vi "Periodic Tasks.vi"(8 "error in":errorcluster) -> ()   [LabVIEW 2015]
doc: "This VI runs in parallel to other tasks. It can contain as many user-defined periodic loops as you need. These can carry out PID or other sorts of timed response."
uses:
  <vilib>/Rock Robotics/WPI/CAN/TalonSRX/WPI_CANTalonSRX_GlobalStatus.ctl
  <vilib>/Rock Robotics/Network Tables/NT Write Number.vi
  <vilib>/Rock Robotics/WPI/Solenoid/Deprecated/WPI_SolenoidSetBool.vi
  <vilib>/Rock Robotics/WPI/Solenoid/Deprecated/WPI_SolenoidGetBool.vi
panel:
  out "LowerRPM":dbl
  out "UpperRPM":dbl
  out "diff":dbl
  out "Talon SRX Status 2":T1
  out "Waveform Chart":cluster{dbl, dbl}(graph)
  in  "dT 2":dbl format="%#_13g"
  in  "I 2":dbl format="%#_13g"
  in  "P 2":dbl=1.0 format="%#_13g"
  in  "dT":dbl format="%#_13g"
  in  "I":dbl format="%#_13g"
  in  "P":dbl=1.0 format="%#_13g"
  out "Talon SRX Status":T1
  out "x/y":dbl=2.0599363125
  out "Shot":bool=TRUE
  in  "Left Art":dbl=0.5 format="%#_13g"
  in  "Right Art":dbl=0.5 format="%#_13g"
  in  "velocity_lower":dbl=1.0 format="%#_13g"
  in  "velocity_upper":dbl=1.0 format="%#_13g"
  out "error out":errorcluster
  # "change in time in milliseconds"
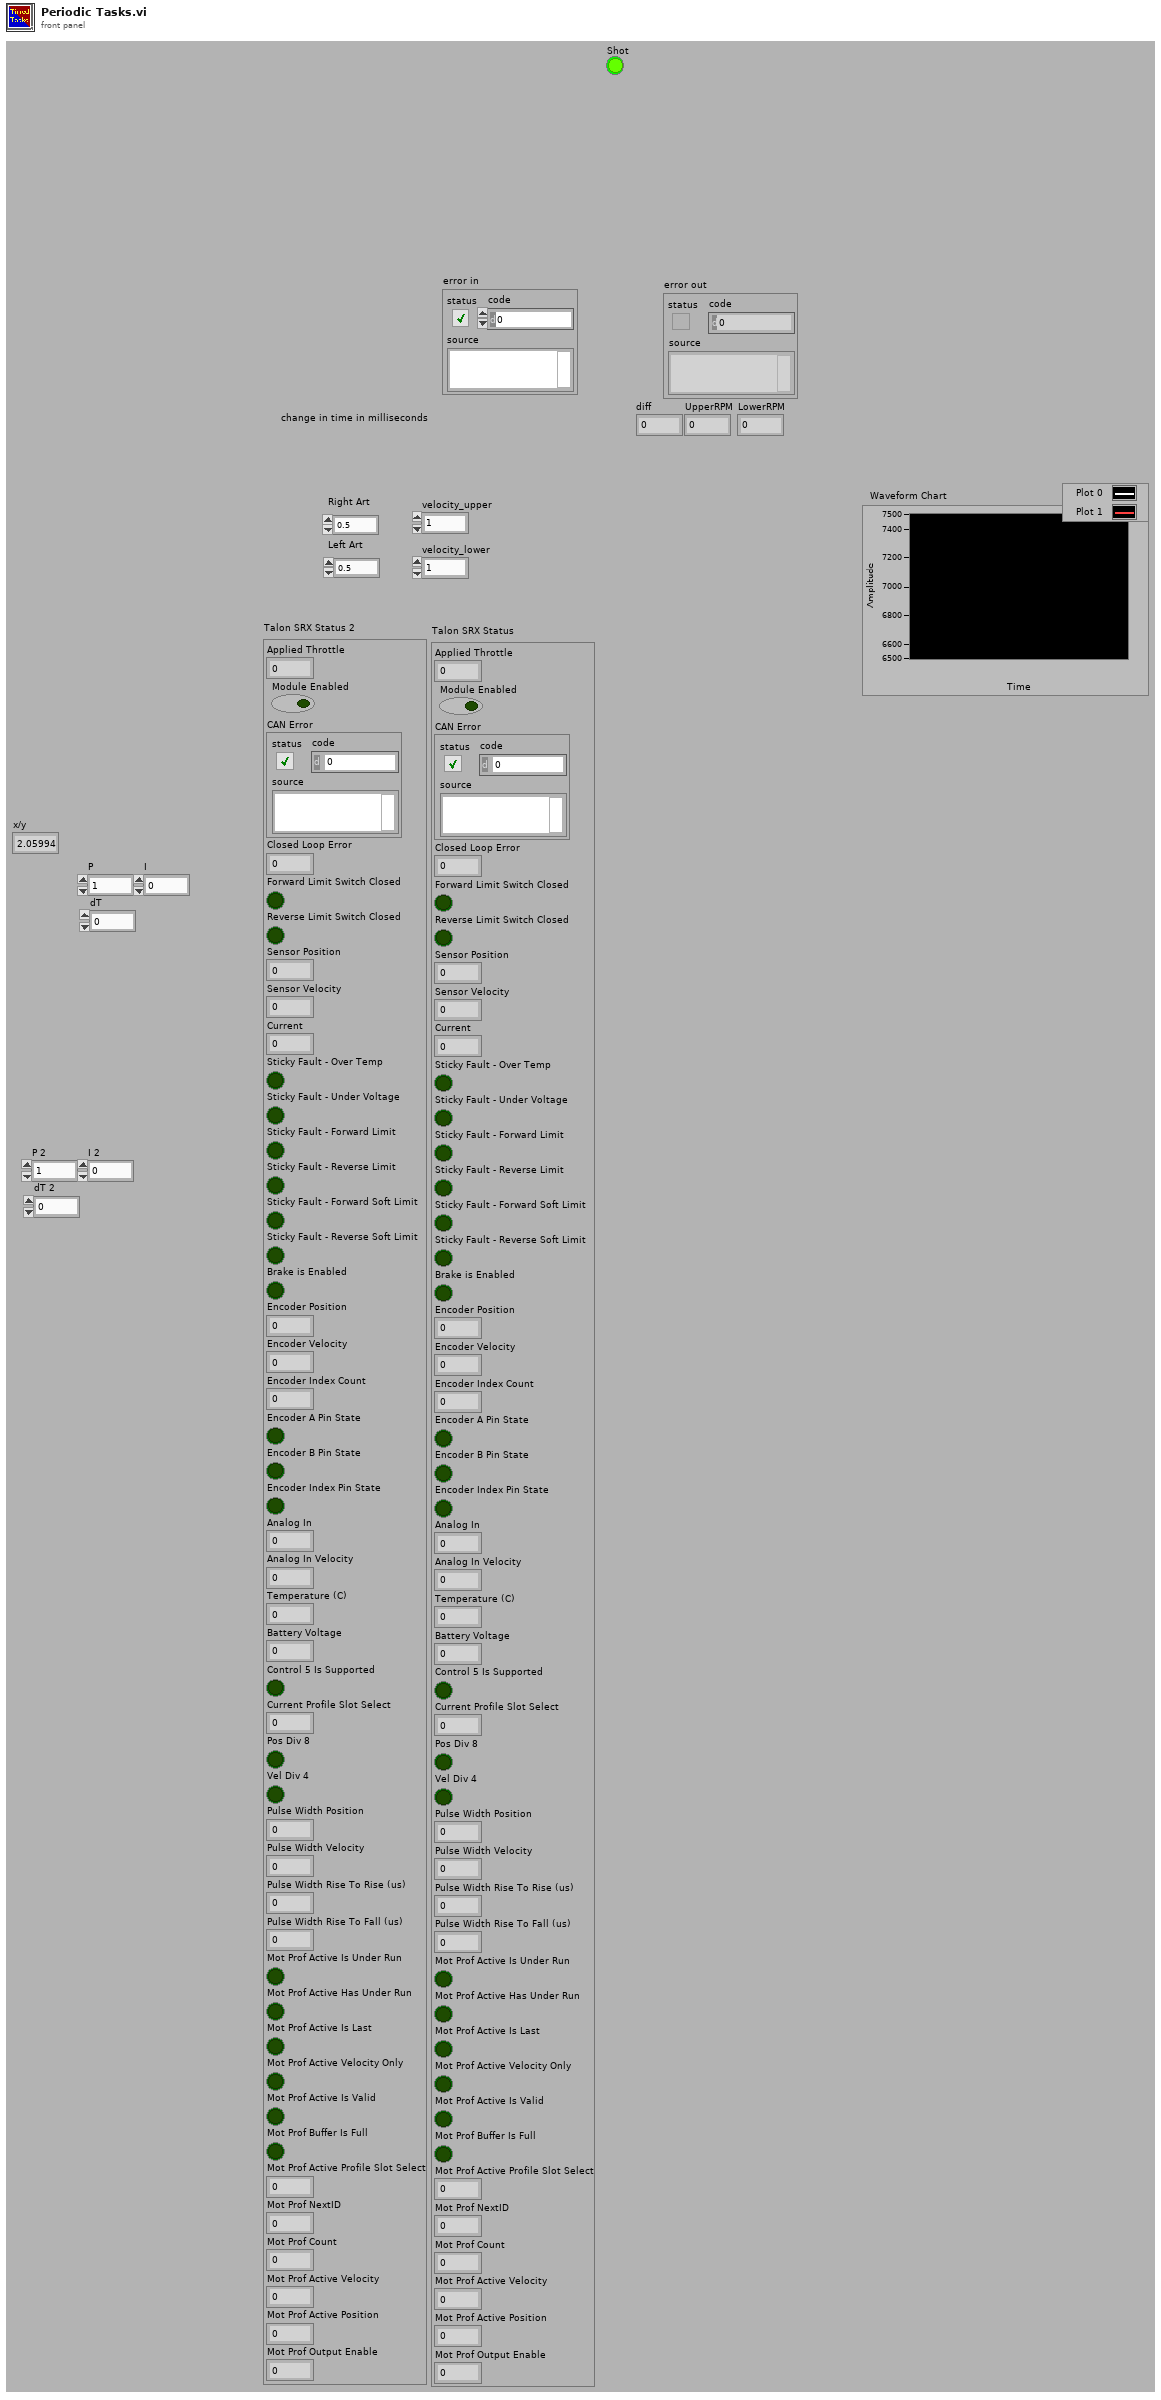
[diagram p1: front panel]
types:
  T1 = typedef "WPI_CANTalonSRX_GlobalStatus.ctl" = cluster{"Applied Throttle":dbl, "Module Enabled":bool, "CAN Error":errorcluster, "Closed Loop Error":dbl, "Forward Limit Switch Closed":bool, "Reverse Limit Switch Closed":bool, "Sensor Position":dbl, "Sensor Velocity":dbl, "Current":dbl, "Sticky Fault - Over Temp":bool, "Sticky Fault - Under Voltage":bool, "Sticky Fault - Forward Limit":bool, "Sticky Fault - Reverse Limit":bool, "Sticky Fault - Forward Soft Limit":bool, "Sticky Fault - Reverse Soft Limit":bool, "Brake is Enabled":bool, "Encoder Position":dbl, "Encoder Velocity":dbl, "Encoder Index Count":dbl, "Encoder A Pin State":bool, "Encoder B Pin State":bool, "Encoder Index Pin State":bool, "Analog In":dbl, "Analog In Velocity":dbl, "Temperature (C)":dbl, "Battery Voltage":dbl, "Control 5 Is Supported":bool, "Current Profile Slot Select":dbl, "Pos Div 8":bool, "Vel Div 4":bool, "Pulse Width Position":i32, "Pulse Width Velocity":i32, "Pulse Width Rise To Rise (us)":i32, "Pulse Width Rise To Fall (us)":i32, "Mot Prof Active Is Under Run":bool, "Mot Prof Active Has Under Run":bool, "Mot Prof Active Is Last":bool, "Mot Prof Active Velocity Only":bool, "Mot Prof Active Is Valid":bool, "Mot Prof Buffer Is Full":bool, "Mot Prof Active Profile Slot Select":i32, "Mot Prof NextID":i32, "Mot Prof Count":i32, "Mot Prof Active Velocity":dbl, "Mot Prof Active Position":dbl, "Mot Prof Output Enable":i32}
  T2 = typedef "WPI_DigitalInputDevRef.ctl" = cluster{"DevStatus":errorcluster, "DIO Channel":T3}
  T3 = typedef "FPGA_DIOChannel.ctl" = enum8{"DIO 0", "DIO 1", "DIO 2", "DIO 3", "DIO 4", "DIO 5", "DIO 6", "DIO 7", "DIO 8", "DIO 9", "DIO MXP 0", "DIO MXP 1", "DIO MXP 2", "DIO MXP 3", "DIO MXP 4", "DIO MXP 5", "DIO MXP 6", "DIO MXP 7", "DIO MXP 8", "DIO MXP 9", "DIO MXP 10", "DIO MXP 11", "DIO MXP 12", "DIO MXP 13", "DIO MXP 14", "DIO MXP 15", "Invalid"}
  T4 = typedef "WPI_MotorControlDeviceRef.ctl" = cluster{"DeviceStatus":errorcluster, "Type":T5, "PWM":cluster{"PWM Channel":T6, "DeadBand":T7}, "CAN":cluster{"Device Number":u8, "Control Mode":T8, "Semaphore":T9, "Max Vout":dbl, "TalonSRX Control Mode":T10}, "Invert":bool}
  T5 = typedef "WPI_MotorControlType.ctl" = enum16{"PWM", "CAN", "CANTalonSRX"}
  T6 = typedef "FPGA_DIOPWMChannel.ctl" = enum8{"PWM 0", "PWM 1", "PWM 2", "PWM 3", "PWM 4", "PWM 5", "PWM 6", "PWM 7", "PWM 8", "PWM 9", "PWM MXP 0", "PWM MXP 1", "PWM MXP 2", "PWM MXP 3", "PWM MXP 4", "PWM MXP 5", "PWM MXP 6", "PWM MXP 7", "PWM MXP 8", "PWM MXP 9", "Invalid"}
  T7 = typedef "WPI_PWMDeadband.ctl" = cluster{"Name":string, "maxPositivePwm":i32, "minPositivePwm":i32, "centerPwm":i32, "maxNegativePwm":i32, "minNegativePwm":i32, "angularRange":u16}
  T8 = typedef "WPI_CANJaguar_ControlMode.ctl" = enum8{"Percent VBus", "Current", "Speed", "Position", "Voltage"}
  T9 = typedef "Semaphore RefNum" = refnum<k1>
  T10 = typedef "WPI_CANTalonSRX_APIControlMode.ctl" = enum8{"Percent VBus", "Speed", "Position", "Slave", "Unchanged / Invalid", "Voltage Compensation", "Current", "Motion Profile"}
  T11 = typedef "WPI_EncoderDevRef.ctl" = cluster{"DevStatus":errorcluster, "EncoderIndex":T12, "CounterIndex":T13, "DistancePerCount":dbl, "Decoding Type":T14}
  T12 = typedef "FPGA_EncoderIdx.ctl" = enum8{"Enc 0", "Enc 1", "Enc 2", "Enc 3", "Enc 4", "Enc 5", "Enc 6", "Enc 7", "Invalid"}
  T13 = typedef "FPGA_CounterCtrSystemIndex.ctl" = enum8{"Ctr 0", "Ctr 1", "Ctr 2", "Ctr 3", "Ctr 4", "Ctr 5", "Ctr 6", "Ctr 7", "Invalid"}
  T14 = typedef "WPI_EncoderType.ctl" = enum16{"1x", "2x", "4x"}
  T15 = typedef "WPI_DriverStationRobotMode2.ctl" = enum16{"Autonomous Disabled", "Autonomous Enabled", "Teleop Disabled", "Teleop Enabled", "Disconnected", "Finish", "Test Disabled", "Test Enabled", "Emergency Stopped"}
  T16 = typedef "WPI_SolenoidDevRef.ctl" = cluster{"DevStatus":errorcluster, "Pneumatics Control Module":u8, "Forward Solenoid Channel":T17, "Reverse Solenoid Channel":T17}
  T17 = typedef "WPI_SolenoidChannel.ctl" = enum8{"Solenoid 0", "Solenoid 1", "Solenoid 2", "Solenoid 3", "Solenoid 4", "Solenoid 5", "Solenoid 6", "Solenoid 7", "Invalid"}
  T18 = typedef "WPI_AnalogChannelDevRef.ctl" = cluster{"DevStatus":errorcluster, "Analog Channel":T19}
  T19 = typedef "FPGA_AIChannel.ctl" = enum8{"AI 0", "AI 1", "AI 2", "AI 3", "AI MXP 0", "AI MXP 1", "AI MXP 2", "AI MXP 3", "Invalid"}
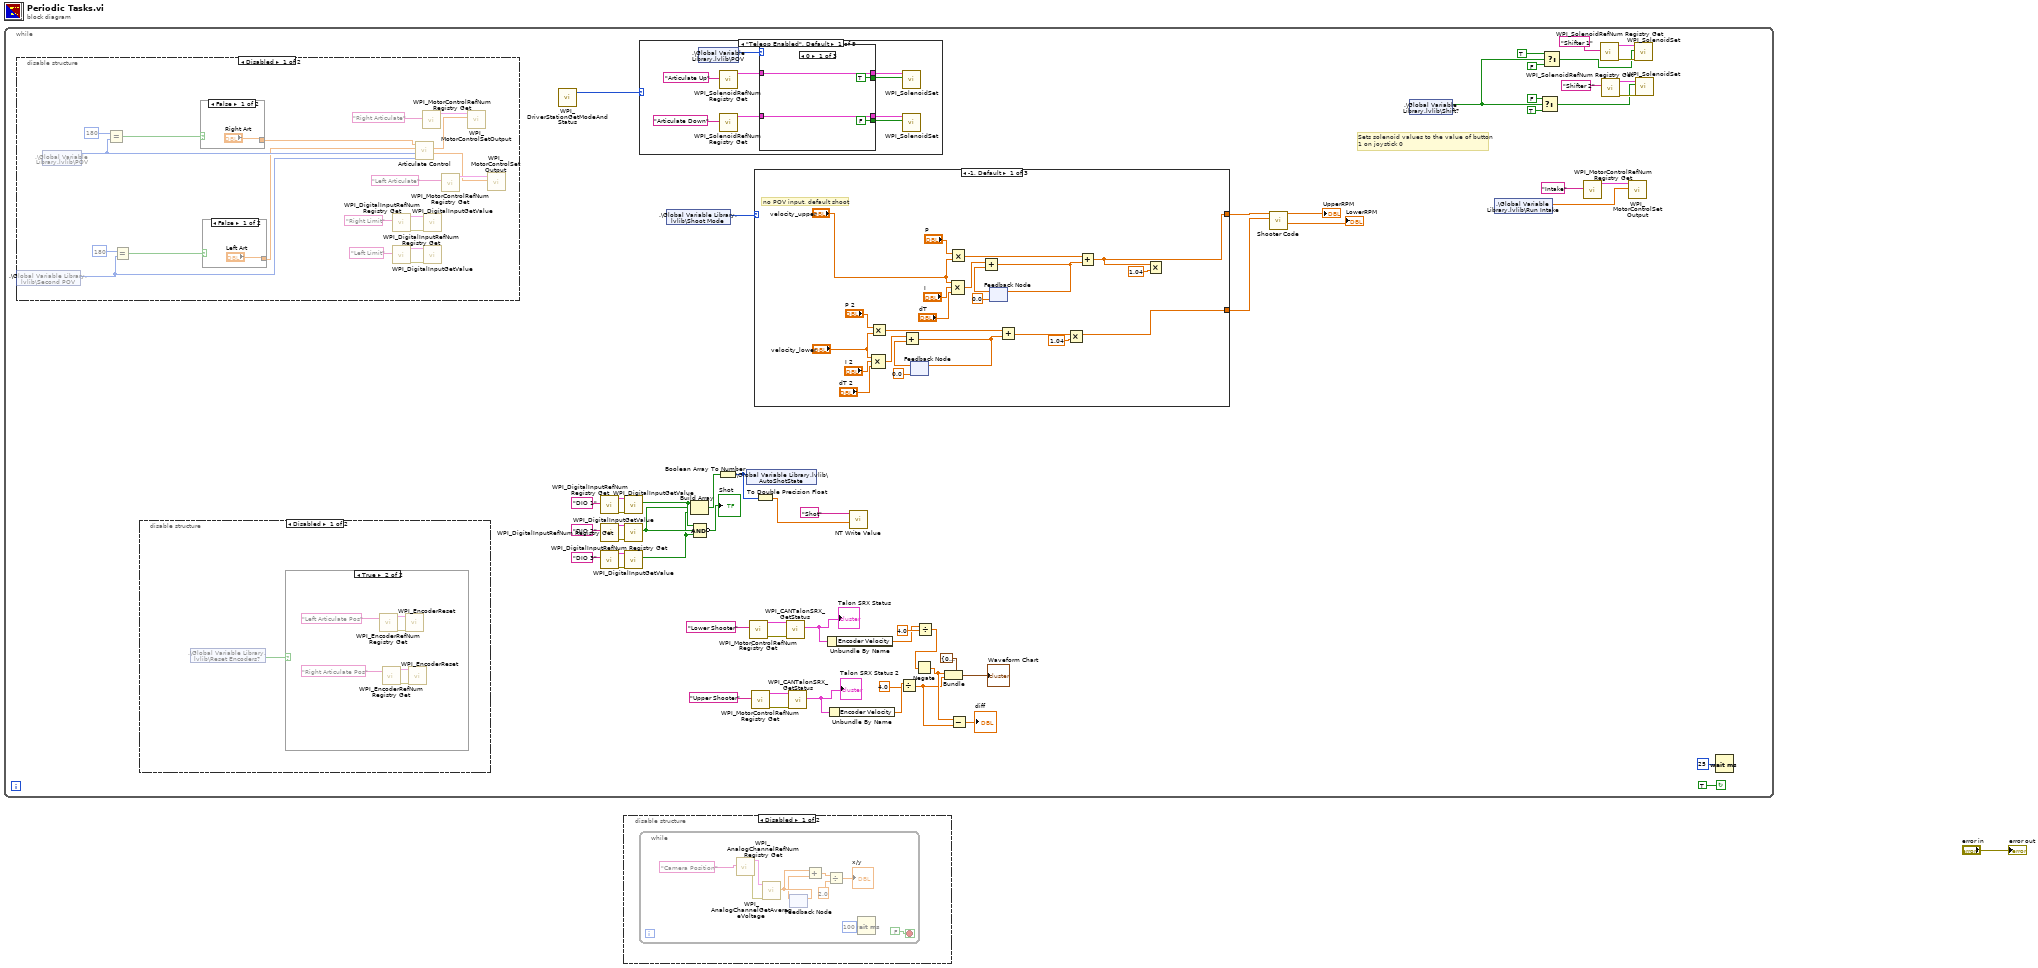
[diagram p0: block diagram]
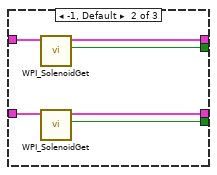
[diagram p3: hidden frame]
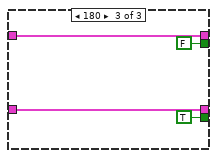
[diagram p4: hidden frame]
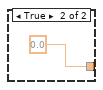
[diagram p15: hidden frame]
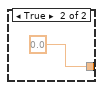
[diagram p16: hidden frame]
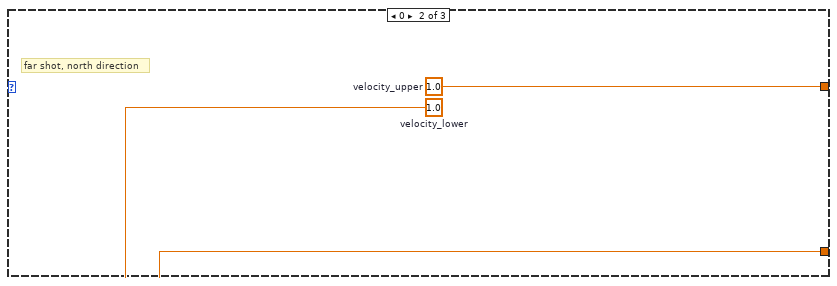
[diagram p18: hidden frame]
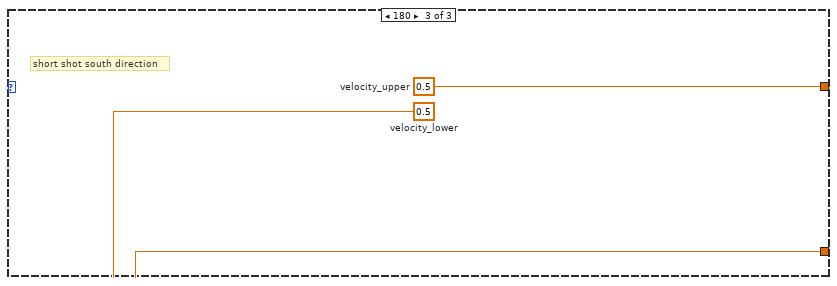
[diagram p19: hidden frame]
diagram:
  n1 = while {
    stop <- TRUE continue-if-true
    # "Sets solenoid values to the value of button\n1 on joystick 0"
    n2 = disable-structure shown="Disabled" {
      frame Disabled {
        n3 = shared-variable ".\\Global Variable Library.lvlib\\Second POV"() -> (w107:i16)  [unwired: 1 in, 1 out]
        n4 = shared-variable ".\\Global Variable Library.lvlib\\POV"() -> (w102:i16)  [unwired: 1 in, 1 out]
        n5 = Equal?(x=i16 180, y=w102) -> (x = y?=w101:bool)
        n6 = Equal?(x=i16 180, y=w107) -> (x = y?=w106:bool)
        n7 = case shown="False" w101 {
          tunnel: ["Right Art" 0.0] -> w103
          frame False {
          }
          frame True {
          }
        }
        n8 = case shown="False" w106 {
          tunnel: ["Left Art" 0.0] -> w97
          frame False {
          }
          frame True {
          }
        }
        n9 = call <vilib>:"WPI_DigitalInputRefNum Registry Get.vi"("refnum name"="Right Limit") -> ("error out"=w91:errorcluster, "DigitalInputDevRef"=w92:T2)  [unwired: 9 in]
        n10 = call <vilib>:"WPI_DigitalInputRefNum Registry Get.vi"("refnum name"="Left Limit") -> ("error out"=w96:errorcluster, "DigitalInputDevRef"=w95:T2)  [unwired: 9 in]
        n11 = call "Articulate Control.vi"("Second POV"=w107, "POV"=w102, "Left Articulate Target"=w97, "Right Articulate Target"=w103) -> ("Left Art Output"=w98:dbl, "Right Art Output"=w105:dbl)  [unwired: 6 in]
        n12 = call <vilib>:"WPI_MotorControlRefNum Registry Get.vi"("refnum name"="Right Articulate") -> ("MotorControlDevRef"=w100:T4)  [unwired: 9 in, 1 out]
        n13 = call <vilib>:"WPI_DigitalInputGetValue.vi"("error in (no error)"=w91, "DigitalInputDevRef"=w92) -> ()  [unwired: 7 in, 3 out]
        n14 = call <vilib>:"WPI_DigitalInputGetValue.vi"("error in (no error)"=w96, "DigitalInputDevRef"=w95) -> ()  [unwired: 7 in, 3 out]
        n15 = call <vilib>:"WPI_MotorControlRefNum Registry Get.vi"("refnum name"="Left Articulate") -> ("MotorControlDevRef"=w109:T4)  [unwired: 9 in, 1 out]
        n16 = call <vilib>:"WPI_MotorControlSetOutput.vi"("Output"=w105, "MotorControlDevRef"=w100) -> ()  [unwired: 7 in, 3 out]
        n17 = call <vilib>:"WPI_MotorControlSetOutput.vi"("Output"=w98, "MotorControlDevRef"=w109) -> ()  [unwired: 7 in, 3 out]
      }
      frame Enabled {
      }
    }
    n18 = disable-structure shown="Disabled" {
      frame Disabled {
        n19 = shared-variable ".\\Global Variable Library.lvlib\\Reset Encoders?"() -> (w84:bool)  [unwired: 1 in, 1 out]
        n20 = case shown="True" w84 {
          frame False {
          }
          frame True {
            n21 = call <vilib>:"WPI_EncoderRefNum Registry Get.vi"("refnum name"="Left Articulate Pos") -> ("error out"=w90:errorcluster, "EncoderDevRef"=w89:T11)  [unwired: 9 in]
            n22 = call <vilib>:"WPI_EncoderRefNum Registry Get.vi"("refnum name"="Right Articulate Pos") -> ("error out"=w85:errorcluster, "EncoderDevRef"=w86:T11)  [unwired: 9 in]
            n23 = call <vilib>:"WPI_EncoderReset.vi"("error in (no error)"=w90, "EncoderDevRef"=w89) -> ()  [unwired: 8 in, 2 out]
            n24 = call <vilib>:"WPI_EncoderReset.vi"("error in (no error)"=w85, "EncoderDevRef"=w86) -> ()  [unwired: 8 in, 2 out]
          }
        }
      }
      frame Enabled {
      }
    }
    n25 = call <vilib>:"WPI_DriverStationGetModeAndStatus.vi"() -> ("Robot Mode"=w39:T15)  [unwired: 10 in, 1 out]
    n26 = call <vilib>:"WPI_DigitalInputRefNum Registry Get.vi"("refnum name"="DIO 1") -> ("error out"=w37:errorcluster, "DigitalInputDevRef"=w36:T2)  [unwired: 9 in]
    n27 = call <vilib>:"WPI_DigitalInputRefNum Registry Get.vi"("refnum name"="DIO 2") -> ("error out"=w34:errorcluster, "DigitalInputDevRef"=w35:T2)  [unwired: 9 in]
    n28 = call <vilib>:"WPI_DigitalInputRefNum Registry Get.vi"("refnum name"="DIO 3") -> ("error out"=w33:errorcluster, "DigitalInputDevRef"=w32:T2)  [unwired: 9 in]
    n29 = call <vilib>:"WPI_DigitalInputGetValue.vi"("error in (no error)"=w37, "DigitalInputDevRef"=w36) -> ("Value"=w26:bool)  [unwired: 7 in, 2 out]
    n30 = call <vilib>:"WPI_DigitalInputGetValue.vi"("error in (no error)"=w34, "DigitalInputDevRef"=w35) -> ("Value"=w25:bool)  [unwired: 7 in, 2 out]
    n31 = call <vilib>:"WPI_DigitalInputGetValue.vi"("error in (no error)"=w33, "DigitalInputDevRef"=w32) -> ("Value"=w24:bool)  [unwired: 7 in, 2 out]
    n32 = case shown="\"Teleop Enabled\", Default" w39 {
      frame "Teleop Enabled", Default {
        n33 = shared-variable ".\\Global Variable Library.lvlib\\POV"() -> (w69:i16)  [unwired: 1 in, 1 out]
        n34 = call <vilib>:"WPI_SolenoidRefNum Registry Get.vi"("refnum name"="Articulate Up") -> ("SolenoidDevRef"=w61:T16)  [unwired: 9 in, 1 out]
        n35 = call <vilib>:"WPI_SolenoidRefNum Registry Get.vi"("refnum name"="Articulate Down") -> ("SolenoidDevRef"=w68:T16)  [unwired: 9 in, 1 out]
        n36 = case shown="0" w69 {
          tunnel: w68 -> [w73 w79 w81]
          tunnel: [w73 w78 w81] -> w67
          tunnel: [FALSE ("Value") w77 TRUE ("Value")] -> w66
          tunnel: w61 -> [w72 w74 w82]
          tunnel: [w72 w75 w82] -> w62
          tunnel: [TRUE ("Value") w76 FALSE ("Value")] -> w63
          frame 0 {
          }
          frame -1, Default {
            n37 = call-poly <vilib>:"WPI_SolenoidGet.vi"("SolenoidDevRef"=w74) -> ("Value"=w76:bool, "SolenoidDevRef"=w75:T16)  [unwired: 8 in, 1 out]
            n38 = call-poly <vilib>:"WPI_SolenoidGet.vi"("SolenoidDevRef"=w79) -> ("Value"=w77:bool, "SolenoidDevRef"=w78:T16)  [unwired: 8 in, 1 out]
          }
          frame 180 {
          }
        }
        n39 = call-poly <vilib>:"WPI_SolenoidSet.vi"("Value"=w63, "SolenoidDevRef"=w62) -> ()  [unwired: 8 in, 2 out]
        n40 = call-poly <vilib>:"WPI_SolenoidSet.vi"("Value"=w66, "SolenoidDevRef"=w67) -> ()  [unwired: 8 in, 2 out]
      }
      frame "Disconnected" {
      }
      frame "Finish" {
      }
      frame "Test Disabled" {
      }
      frame "Test Enabled" {
      }
      frame "Emergency Stopped" {
      }
      frame "Teleop Disabled" {
      }
      frame "Autonomous Enabled" {
      }
      frame "Autonomous Disabled" {
      }
    }
    n41 = shared-variable ".\\Global Variable Library.lvlib\\Shoot Mode"() -> (w41:i16)  [unwired: 1 in, 1 out]
    n42 = Build Array(w26, w25, w24) -> (w27:bool[])
    n43 = Compound Arithmetic op=AND(w26, w25, w24) -> (invert →"Shot":bool)
    n44 = Boolean Array To Number(Boolean array=w27) -> (number=w23:u32)
    n45 = shared-variable ".\\Global Variable Library.lvlib\\AutoShotState"(w23) -> ()  [unwired: 1 in, 1 out]
    n46 = call <vilib>:"WPI_MotorControlRefNum Registry Get.vi"("refnum name"="Lower Shooter") -> ("error out"=w21:errorcluster, "MotorControlDevRef"=w20:T4)  [unwired: 9 in]
    n47 = call <vilib>:"WPI_MotorControlRefNum Registry Get.vi"("refnum name"="Upper Shooter") -> ("error out"=w14:errorcluster, "MotorControlDevRef"=w15:T4)  [unwired: 9 in]
    n48 = case shown="-1, Default" w41 {
      tunnel: [w127 w138 w140] -> w43
      tunnel: [w117 w137 w139] -> w42
      frame -1, Default {
        # "no POV input, default shoot"
        n49 = Multiply(x="P 2", y="velocity_lower") -> (x*y=w126:dbl)
        n50 = Compound Arithmetic op=MULTIPLY("velocity_lower", "I 2", "dT 2") -> (w119:dbl)
        n51 = feedback #1(0.0) -> (w120:dbl)
        n52 = Add(x=w119, y=w120) -> (x+y=w121:dbl)
        n53 = feedback-in #1(w121) -> ()
        n54 = Multiply(x="P", y="velocity_upper") -> (x*y=w136:dbl)
        n55 = Compound Arithmetic op=MULTIPLY("velocity_upper", "I", "dT") -> (w129:dbl)
        n56 = feedback #2(0.0) -> (w130:dbl)
        n57 = Add(x=w129, y=w130) -> (x+y=w131:dbl)
        n58 = feedback-in #2(w131) -> ()
        n59 = Add(x=w126, y=w121) -> (x+y=w117:dbl)
        n60 = Multiply(x=w117, y=1.04) -> ()  [unwired: 1 out]
        n61 = Add(x=w136, y=w131) -> (x+y=w127:dbl)
        n62 = Multiply(x=w127, y=1.04) -> ()  [unwired: 1 out]
      }
      frame 0 {
        w137 = 1.0  # velocity_lower
        w138 = 1.0  # velocity_upper
        # "far shot, north direction"
      }
      frame 180 {
        w139 = 0.5  # velocity_lower
        w140 = 0.5  # velocity_upper
        # "short shot south direction"
      }
    }
    n63 = To Double Precision Float(number=w23) -> (double precision float=w22:dbl)
    n64 = call <vilib>:"WPI_CANTalonSRX_GetStatus.vi"("error in (no error)"=w21, "CAN Talon SRX Ref"=w20) -> ("Talon SRX Status"=w18:T1)  [unwired: 7 in, 2 out]
    "Talon SRX Status" <- w18
    n65 = call <vilib>:"WPI_CANTalonSRX_GetStatus.vi"("error in (no error)"=w14, "CAN Talon SRX Ref"=w15) -> ("Talon SRX Status"=w17:T1)  [unwired: 7 in, 2 out]
    "Talon SRX Status 2" <- w17
    n66 = Unbundle By Name(w18) -> ("Encoder Velocity"=w7:dbl)
    n67 = Unbundle By Name(w17) -> ("Encoder Velocity"=w10:dbl)
    n68 = call-poly <vilib>:"NT Write Value.vi"("Numeric"=w22, "Name"="Shot") -> ()  [unwired: 9 in, 1 out]
    n69 = Divide(x=w10, y=4.0) -> (x/y=w5:dbl)
    n70 = Divide(x=w7, y=4.0) -> (x/y=w11:dbl)
    n71 = Negate(x=w11) -> (-x=w6:dbl)
    n72 = Bundle(cluster=cluster{dbl, dbl} {0.0, 0.0}, w6, w5) -> (→"Waveform Chart":cluster{dbl, dbl})
    n73 = Subtract(x=w6, y=w5) -> (x-y=→"diff":dbl)
    n74 = call "Shooter Code.vi"("velocity_lower"=w42, "velocity_upper"=w43) -> ("lowerRPM"=→"LowerRPM":dbl, "upperRPM"=→"UpperRPM":dbl)  [unwired: 8 in]
    n75 = shared-variable ".\\Global Variable Library.lvlib\\Shift?"() -> (w46:bool)  [unwired: 1 in, 1 out]
    n76 = shared-variable ".\\Global Variable Library.lvlib\\Run Intake"() -> (w40:dbl)  [unwired: 1 in, 1 out]
    n77 = Select(t=FALSE ("f"), s=w46, f=TRUE) -> (s? t:f=w47:bool)
    n78 = Select(t=TRUE, s=w46, f=FALSE) -> (s? t:f=w48:bool)
    n79 = call <vilib>:"WPI_MotorControlRefNum Registry Get.vi"("refnum name"="Intake") -> ("MotorControlDevRef"=w44:T4)  [unwired: 9 in, 1 out]
    n80 = call <vilib>:"WPI_SolenoidRefNum Registry Get.vi"("refnum name"="Shifter 1") -> ("error out"=w56:errorcluster, "SolenoidDevRef"=w55:T16)  [unwired: 9 in]
    n81 = call <vilib>:"WPI_SolenoidRefNum Registry Get.vi"("refnum name"="Shifter 2") -> ("error out"=w54:errorcluster, "SolenoidDevRef"=w53:T16)  [unwired: 9 in]
    n82 = call <vilib>:"WPI_MotorControlSetOutput.vi"("Output"=w40, "MotorControlDevRef"=w44) -> ()  [unwired: 7 in, 3 out]
    n83 = call-poly <vilib>:"WPI_SolenoidSet.vi"("error in (no error)"=w56, "Value"=w48, "SolenoidDevRef"=w55) -> ()  [unwired: 7 in, 2 out]
    n84 = call-poly <vilib>:"WPI_SolenoidSet.vi"("error in (no error)"=w54, "Value"=w47, "SolenoidDevRef"=w53) -> ()  [unwired: 7 in, 2 out]
    n85 = Wait (ms)(milliseconds to wait=u32 25) -> ()  [unwired: 1 out]
  }
  n86 = disable-structure shown="Disabled" {
    frame Disabled {
      n87 = while {
        stop <- FALSE stop-if-true
        n88 = call <vilib>:"WPI_AnalogChannelRefNum Registry Get.vi"("refnum name"="Camera Position") -> ("error out"=w145:errorcluster, "AIDeviceRef"=w144:T18)  [unwired: 9 in]
        n89 = call <vilib>:"WPI_AnalogChannelGetAverageVoltage.vi"("error in (no error)"=w145, "AIDeviceRef"=w144) -> ("Voltage"=w147:dbl)  [unwired: 7 in, 2 out]
        n90 = feedback #3() -> (w146:dbl)  [unwired: 1 in]
        n91 = feedback-in #3(w147) -> ()
        n92 = Add(x=w147, y=w146) -> (x+y=w148:dbl)
        n93 = Divide(x=w148, y=2.0) -> (x/y=→"x/y":dbl)
        n94 = Wait (ms)(milliseconds to wait=100) -> ()  [unwired: 1 out]
      }
    }
    frame Enabled {
    }
  }
  "error out" <- "error in"
